vi "Start_Stop.vi"() -> (7 "Command Line Output":string)   [LabVIEW 2018]
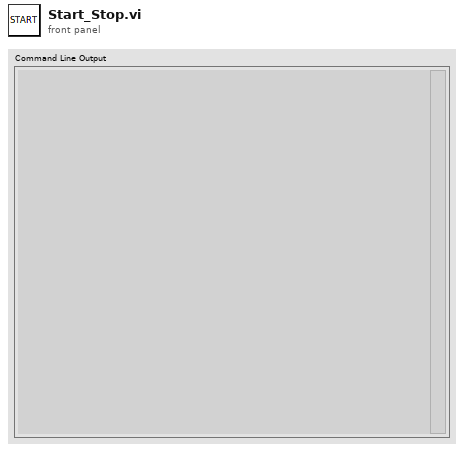
[diagram p1: front panel]
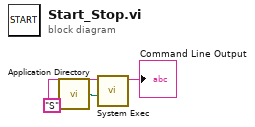
[diagram p0: block diagram]
diagram:
  n1 = call <vilib>:"Application Directory.vi"() -> ("Application Directory"=w1:path)
  n2 = call <vilib>:"System Exec.vi"("working directory"=w1, "command line"="S" ("Start/Stop")) -> ("standard output"=→"Command Line Output":string)  [unwired: 6 in, 3 out]
